vi "Read Discrete Inputs Response.vi"(8 "error in (no error)":errorcluster, 10 "Modbus data unit in":refnum<class "Modbus Data Unit (PDU).lvclass">) -> (0 "error out":errorcluster, 2 "data":bool[](array[boolean]))   [LabVIEW 2020, in "SubVIs.lvlib" / "Master Function Definition.lvlib"]
doc: "Decodes the response for the read discrete inputs function."
uses:
  <vilib>/Modbus/subvis/Data and Functions/Master Function Definition/Master Function Definition.lvlib
  <vilib>/Modbus/subvis/Modbus Data Unit (PDU)/Modbus Data Unit (PDU).lvclass
  <vilib>/Modbus/subvis/SubVIs.lvlib
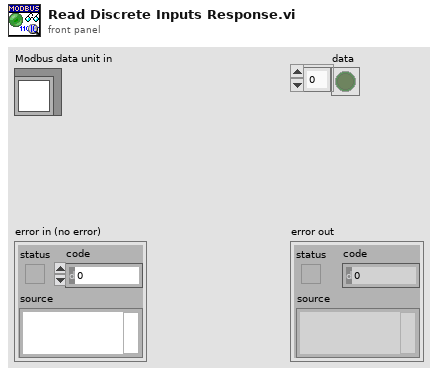
[diagram p1: front panel]
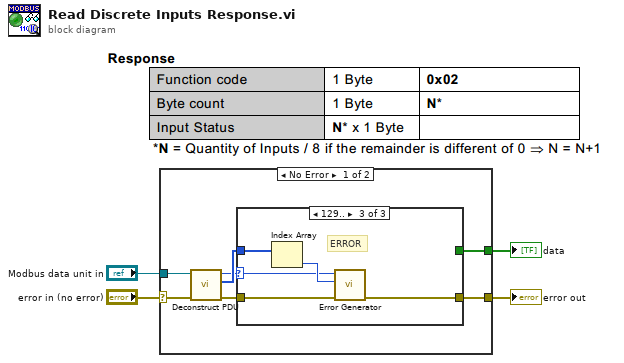
[diagram p0: block diagram]
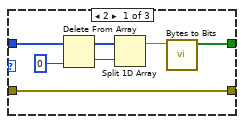
[diagram p2: hidden frame]
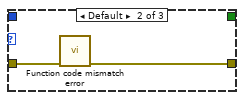
[diagram p3: hidden frame]
diagram:
  n1 = case shown="No Error" "error in (no error)" {
    selector: "error in (no error)" -> [w9 w26]
    tunnel: [w11 w26] -> w3
    tunnel: "Modbus data unit in" -> [w7 _]
    tunnel: [w10 _] -> w1
    frame No Error {
      n2 = call <vilib>:"Deconstruct PDU.vi"("error in (no error)"=w9, "Modbus data unit in"=w7) -> ("error out"=w6:errorcluster, "data"=w8:u8[], "function"=w5:u8)  [unwired: 7 in]
      n3 = case shown="129.." w5 {
        selector: w5 -> [_ _ w21]
        tunnel: w6 -> [w16 w20 w22]
        tunnel: w8 -> [w18 _ w25]
        tunnel: [w16 w19 w24] -> w11
        tunnel: [w17 _ _] -> w10
        frame 2 {
          n4 = Delete From Array(array=w18, index=0) -> (deleted portion=w13:u8, array with subset deleted=w12:u8[])  [unwired: 1 in]
          n5 = Split 1D Array(array=w12, index=w13) -> (first subarray=w15:u8[])  [unwired: 1 out]
          n6 = call <vilib>:"Bytes to Bits.vi"("bytes"=w15) -> ("bits"=w17:bool[])  [unwired: 10 in]
        }
        frame Default {
          n7 = call <vilib>:"Function code mismatch error.vi"("error in (no error)"=w20) -> ("error out"=w19:errorcluster)  [unwired: 10 in]
        }
        frame 129.. {
          # "ERROR"
          n8 = Index Array(array=w25) -> (element=w23:u8)  [unwired: 1 in]
          n9 = call <vilib>:"Error Generator.vi"("error in (no error)"=w22, "data return (error code)"=w23, "function return"=w21) -> ("error out"=w24:errorcluster)  [unwired: 8 in]
        }
      }
    }
    frame Error {
    }
  }
  "error out" <- w3
  "data" <- w1
